vi "test_Copy Slot.vi"(8 "error in (no error)":errorcluster, 11 "TestCase in":refnum<class "Scan Engine Scripting API Custom Device Unit Tests.lvclass">) -> (0 "error out":errorcluster, 3 "TestCase out":refnum<class "Scan Engine Scripting API Custom Device Unit Tests.lvclass">)   [LabVIEW 2019, in "Scan Engine Scripting API Custom Device Unit Tests.lvclass"]
uses:
  Scan Engine Scripting API Custom Device Unit Tests.lvclass
  Type Defs/Local Chassis Settings.ctl
  Scripting/Modules/Mode Classes/Counter Driven Output Mode/Drive from Slot.ctl
  Scripting/Modules/NI 9474/NI 9474.lvclass
  C:/Users/nitest/Desktop/Git 2019/niveristand-scan-engine-ethercat-custom-device/Custom Device Source/Scripting/Modules/Module/Module.lvclass
  Scan Engine Scripting API Custom Device Unit Tests.lvclass/Scan Engine Scripting API Custom Device Unit Tests.ctl
  Type Defs/Main Settings.ctl
  c7e83f66-a965-41fd-b07a-d8c29414f51e.vi
  a134009e-d5c9-407c-b835-1c4aa24009a3.vi
  Utility/Set Error.vi
  <vilib>/Utility/error.llb/Clear Errors.vi
  Scripting/Utility/Convert Slot Configuration to 9212.vi
  Scripting/Utility/Convert Slot Configuration to 9213.vi
  Modules.lvlibp/SD Module/SD Module.lvclass
  C:/Users/nitest/Desktop/Git 2019/niveristand-scan-engine-ethercat-custom-device/Custom Device Source/Modules.lvlibp/RSI Module/RSI Module.lvclass
  Scripting/Modules/NI 9212/NI 9212.lvclass
  Scripting/Modules/NI 9213/NI 9213.lvclass
  Scripting/Modules/NI 9224/NI 9224.lvclass
  Scripting/Modules/NI 9228/NI 9228.lvclass
  Modules.lvlibp/RSI Module/Read Module Page Property.vi
  Modules.lvlibp/RSI Module/Read Model.vi
  Scripting/Utility/Convert Module Model to Module Class.vi
  Modules.lvlibp/SD Module/Read DIO mode.vi
  Modules.lvlibp/RSI Module/Read Channels.vi
  Scripting/Utility/Convert to DI Module.vi
  Scripting/Utility/Convert to DO Module.vi
  Scripting/Utility/Convert to CI PWM Module.vi
  Scripting/Utility/Convert to CDO Module.vi
  Scripting/Utility/Convert to PWM Module.vi
  Globals/Error Strings.vi
  Scripting/Utility/Get Channel Names and Default Values for Slot.vi
  Scripting/Modules/NI 9212/Create NI 9212.vi
  Scripting/Modules/NI 9213/Create NI 9213.vi
  Scripting/Utility/Convert to AI Module.vi
  Scripting/Utility/Convert to AI Vrms Module.vi
  Scripting/Utility/Convert to AI Arms Module.vi
  Scripting/Utility/Convert to DIO Module.vi
  Scripting/Modules/Module/Module.lvclass
  Modules.lvlibp/9212/9212.lvclass
  Modules.lvlibp/9213/9213.lvclass
  Modules.lvlibp/9224/9224.lvclass
  <vilib>/addons/_JKI Toolkits/VI Tester/TestCase.llb/TestCase.lvclass
  Scripting/Scan Engine Scripting.lvlib
  Scan Engine Custom Device.lvlib
  Scripting/Modules/Mode Classes/Counter Driven Output Mode/Counter Driven Output Mode.lvclass
  C:/Program Files (x86)/National Instruments/LabVIEW 2019/vi.lib/addons/_JKI Toolkits/VI Tester/TestCase.llb/TestCase.lvclass
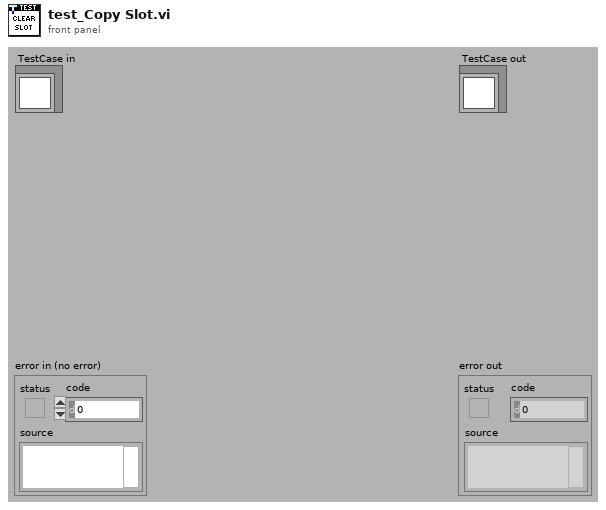
[diagram p1: front panel]
types:
  T1 = typedef "Scan Engine Scripting.lvlib/Counter Driven Output Mode.lvclass/Drive from Slot.ctl" = enum16{"Slot 1", "Slot 2", "Slot 3", "Slot 4", "Slot 5", "Slot 6", "Slot 7", "Slot 8"}
  T2 = typedef "Scan Engine Custom Device.lvlib/Local Chassis Settings.ctl" = cluster{"name":string, "number of slots":i32}
  T3 = typedef "Scan Engine Custom Device.lvlib/Main Settings.ctl" = cluster{"sync to scan":bool, "scan engine decimation":u16, "delay after FPGA load (s)":u16}
  T4 = typedef "Custom Device API.lvlib/Custom Device Item Ref.ctl" = u64
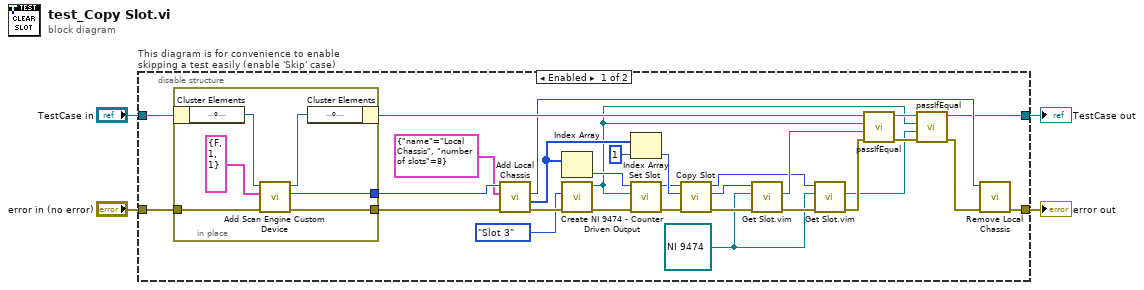
[diagram p0: block diagram]
diagram:
  n1 = disable-structure "This diagram is for convenience to enable skipping a test easily (enable 'Skip' case)" shown="Enabled" {
    disable-tunnel: "TestCase in" -> [w31 w44]
    disable-tunnel: [w11 w42] -> w1
    disable-tunnel: [w19 w43] -> w3
    disable-tunnel: "error in (no error)" -> [w32 w41]
    frame Enabled {
      w9 = refnum<class "NI 9474.lvclass"> refnum ("NI 9474 out")
      n2 = in-place {
        in-place-border: [w40] -> w34
        in-place-border: [w39] -> w33
        in-place-border: w32 -> [w37]
        n3 = in-place-cluster #1(w31) -> ("target ref"=w36:refnum<k24>)
        n4 = call "Add Scan Engine Custom Device.vi"("error in"=w37, "settings"=T3 {"sync to scan"=FALSE, "scan engine decimation"=1, "delay after FPGA load (s)"=1}, "target in"=w36) -> ("error out"=w39:errorcluster, "scan engine custom device ref"=w40:T4, "target out"=w35:refnum<k24>)  [unwired: 6 in]
        n5 = in-place-cluster #1("target ref"=w35) -> (w30:refnum<class "Scan Engine Scripting API Custom Device Unit Tests.lvclass">)
      }
      n6 = call "Add Local Chassis.vi"("error in"=w33, "settings"=T2 {"name"="Local Chassis", "number of slots"=8}, "scan engine custom device ref in"=w34) -> ("error out"=w27:errorcluster, "slot refs"=w24:T4[], "local chassis ref"=w29:T4)  [unwired: 4 in, 2 out]
      n7 = Index Array(array=w24) -> (element=w23:T4)  [unwired: 1 in]
      n8 = call "Create NI 9474 - Counter Driven Output.vi"("error in"=w27, "drive from slot"=Drive_from_Slot."Slot 3") -> ("error out"=w26:errorcluster, "NI 9474 out"=w6:refnum<class "NI 9474.lvclass">)  [unwired: 8 in]
      n9 = Index Array(array=w24, index=1) -> (element=w22:T4)
      n10 = call "Set Slot.vi"("error in"=w26, "module"=w6, "slot ref in"=w23) -> ("error out"=w28:errorcluster, "slot ref out"=w15:T4)  [unwired: 7 in]
      n11 = call "Copy Slot.vi"("error in"=w28, "destination slot ref in"=w22, "source slot ref in"=w15) -> ("error out"=w21:errorcluster, "destination slot ref out"=w7:T4, "source slot ref out"=w8:T4)  [unwired: 6 in]
      n12 = call "Get Slot.vim"("error in"=w21, "module type"=w9, "slot ref in"=w7) -> ("error out"=w20:errorcluster, "module"=w17:refnum<class "NI 9474.lvclass">)  [unwired: 5 in, 2 out]
      n13 = call "Get Slot.vim"("error in"=w20, "module type"=w9, "slot ref in"=w8) -> ("error out"=w18:errorcluster, "module"=w10:refnum<class "NI 9474.lvclass">)  [unwired: 5 in, 2 out]
      n14 = call-dynamic "passIfEqual.vi"("error in (no error)"=w18, "y"=w17, "x"=w6, "TestCase in"=w30) -> ("error out"=w16:errorcluster, "TestCase out"=w12:refnum<class "Scan Engine Scripting API Custom Device Unit Tests.lvclass">)  [unwired: 6 in]
      n15 = call-dynamic "passIfEqual.vi"("error in (no error)"=w16, "y"=w10, "x"=w6, "TestCase in"=w12) -> ("error out"=w13:errorcluster, "TestCase out"=w11:refnum<class "Scan Engine Scripting API Custom Device Unit Tests.lvclass">)  [unwired: 6 in]
      n16 = call "Remove Local Chassis.vi"("error in"=w13, "local chassis ref"=w29) -> ("error out"=w19:errorcluster)  [unwired: 9 in]
    }
    frame Disabled {
      # "skip test result while test is under development"
      n17 = call <vilib>:"skip.vi"("error in (no error)"=w41, "TestCase in"=w44) -> ("error out"=w43:errorcluster, "TestCase out"=w42:refnum<class "Scan Engine Scripting API Custom Device Unit Tests.lvclass">)  [unwired: 8 in]
    }
  }
  "error out" <- w3
  "TestCase out" <- w1
